vi "Receive Message.vi"(6 "priority":i32, 10 "Topic in":refnum<class "Topic.lvclass">, 11 "Message in":refnum<class "Message.lvclass">) -> (0 "error out":errorcluster, 2 "Actor out":refnum<class "Actor.lvclass">)   [LabVIEW 2017, in "Mediator.lvlib" / "Topic.lvclass"]
doc: "This VI should be overriden ONLY if you are creating a proxy actor for remote transmission. If you are, override this VI to transmit the received message to a new destination, maintaining the given priority."
uses:
  Topic.lvclass
  <vilib>/ActorFramework/Message/Message.lvclass
  <vilib>/ActorFramework/Actor/Actor.lvclass
  Topic Messages/Notify Subscribers Msg/Notify Subscribers Msg.lvclass
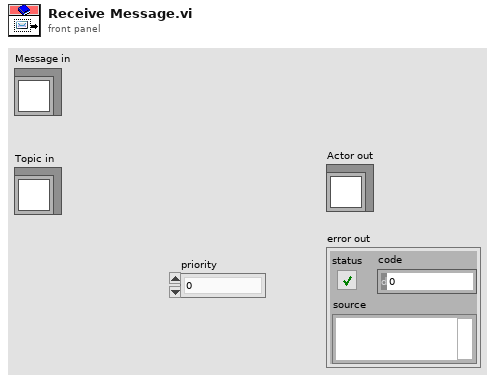
[diagram p1: front panel]
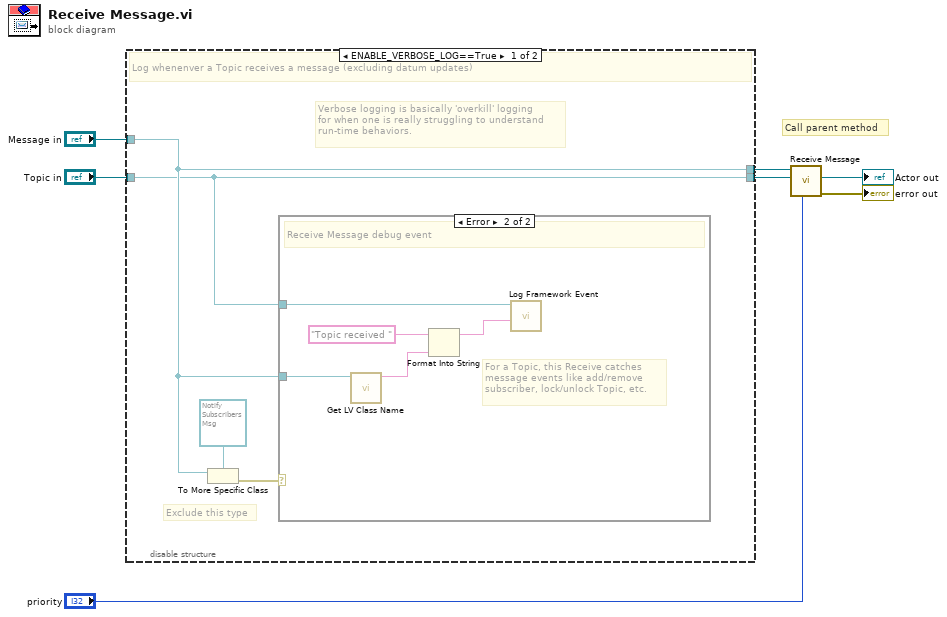
[diagram p0: block diagram]
diagram:
  # "Call parent method"
  n1 = disable-structure shown="ENABLE_VERBOSE_LOG==True" {
    disable-tunnel: "Message in" -> [w11 w18]
    disable-tunnel: "Topic in" -> [w8 w17]
    disable-tunnel: [w11 w18] -> w2
    disable-tunnel: [w8 w17] -> w1
    frame condition #0 {
      # "Verbose logging is basically 'overkill' logging\nfor when one is really struggling to understand\nrun-time behaviors."
      # "Exclude this type"
      # "Log whenenver a Topic receives a message (excluding datum updates)"
      n2 = To More Specific Class(target class=refnum<class "Notify Subscribers Msg.lvclass"> refnum ("Mediator.lvlib:Notify Subscribers Msg.lvclass"), reference=w11) -> (error out=w9:errorcluster)  [unwired: 1 in, 1 out]
      n3 = case shown="Error" w9 {
        tunnel: w11 -> [_ w15]
        tunnel: w8 -> [_ w16]
        frame No Error {
          # "Exclude logging for mediated datum updates\nbecause there are just too many of them.\n\n(The MediatorBusMonitor provides this information\nby showing all data bus updates in real time.)"
          # "Message is a Notify Subscribers Msg -- Do not log this message type"
        }
        frame Error {
          # "For a Topic, this Receive catches\nmessage events like add/remove\nsubscriber, lock/unlock Topic, etc."
          # "Receive Message debug event"
          n4 = call <vilib>:"Get LV Class Name.vi"("object"=w15) -> ("class name"=w13:string)  [unwired: 9 in, 1 out]
          n5 = Format Into String(initial string="Topic received ", w13) -> (resulting string=w12:string)  [unwired: 2 in, 1 out]
          n6 = call "Log Framework Event.vi"("Data To Log"=w12, "Topic In"=w16) -> ()  [unwired: 9 in, 1 out]
        }
      }
    }
    frame condition #1 (active) {
      # "Remove all logging from this method at compile time"
    }
  }
  n7 = call-parent "Receive Message.vi"("priority"="priority", "Actor in"=w1, "Message in"=w2) -> ("error out"=→"error out":errorcluster, "Actor out"=→"Actor out":refnum<class "Actor.lvclass">)  [unwired: 7 in]
